vi "Storing Calibration Coefficients.vi"(11 "output cluster":T1) -> (1 "Array":dbl[](array[numeric]), 2 "Error":bool)   [LabVIEW 2016]
uses:
  Controls/Cal Refs.ctl
  Miscellaneous/Globals.vi
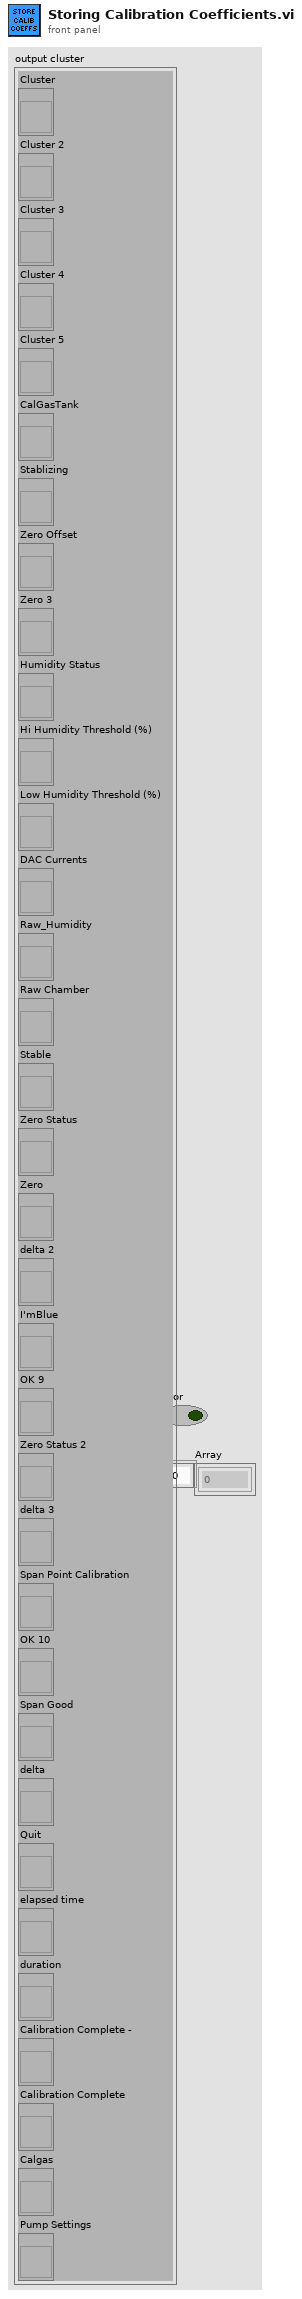
[diagram p1: front panel]
types:
  T1 = typedef "Cal Refs.ctl" = cluster{"Cluster":refnum<vi>, "Cluster 2":refnum<vi>, "Cluster 3":refnum<vi>, "Cluster 4":refnum<vi>, "Cluster 5":refnum<vi>, "CalGasTank":refnum<vi>, "Stablizing":refnum<vi>, "Zero Offset":refnum<vi>, "Zero 3":refnum<vi>, "Humidity Status":refnum<vi>, "Hi Humidity Threshold (%)":refnum<vi>, "Low Humidity Threshold (%)":refnum<vi>, "DAC Currents":refnum<vi>, "Raw_Humidity":refnum<vi>, "Raw Chamber":refnum<vi>, "Stable":refnum<vi>, "Zero Status":refnum<vi>, "Zero":refnum<vi>, "delta 2":refnum<vi>, "I'mBlue":refnum<vi>, "OK 9":refnum<vi>, "Zero Status 2":refnum<vi>, "delta 3":refnum<vi>, "Span Point Calibration":refnum<vi>, "OK 10":refnum<vi>, "Span Good":refnum<vi>, "delta":refnum<vi>, "Quit":refnum<vi>, "elapsed time":refnum<vi>, "duration":refnum<vi>, "Calibration Complete -":refnum<vi>, "Calibration Complete":refnum<vi>, "Calgas":refnum<vi>, "Pump Settings":refnum<vi>}
  T2 = typedef "Calibration Coefficients.ctl" = cluster{"CalFile Used":path, "TYPE":string, "DATE":string, "Humidity":sgl, "Chamber Temp":dbl, "CO2_calgas":dbl, "V_(RA,5mA)":dbl, "V_(RA,15mA)":dbl, "mI":dbl, "V_0d_ImA (actual)":dbl, "V_6d_ImA (actual)":dbl, "I_span":dbl, "DAC":u16, "A":dbl, "B":dbl, "C":dbl, "D":dbl, "V6d":dbl, "A'":dbl, "B'":dbl, "C'":dbl, "D'":dbl, "V0d":dbl, "CalDate":string, "CalTime":string, "duration":dbl, "Detector Channel":string, "a2":dbl, "a3":dbl, "a4":dbl, "a5":dbl, "b2":dbl, "c2":dbl, "b3":dbl, "c3":dbl, "b4":dbl, "c4":dbl, "b5":dbl, "c5":dbl, "a7":dbl, "a8":dbl, "a9":dbl, "a10":dbl, "b7":dbl, "b8":dbl, "b9":dbl, "b10":dbl, "c7":dbl, "c8":dbl, "c9":dbl, "c10":dbl, "cal_offs_adj":dbl, "cal_gain_adj":dbl, "C6d":dbl, "C0d":dbl, "Cal_currernt":dbl, "C2V":u16, "V2C":u16, "Zero Date":string, "Zero Time":string, "Number of Zeroes":u16, "V_(()d, average)":dbl, "V_offs ":dbl, "G_adj":dbl, "Pump Flow Rate":u16, "Zero Required? ":bool, "Calibrate Required?":bool, "cal_utc":dbl, "zero_utc":dbl, "Elapsed Time":dbl, "PCB":string, "m0":dbl, "b0":dbl}
  T3 = cluster{"CalFile Selected":path, "TYPE":string, "DATE":string, "C0FC2V":dbl[], "C6FC2V":dbl[], "V_0d(target)":dbl[], "V_6d(target)":dbl[], "V_span(target)":dbl[], "CHANNEL":string[], "Status":bool[], "BlueLED 2":bool[], "C2V":u8[], "A":dbl[], "B":dbl[], "C":dbl[], "D":dbl[], "V2C":u8[], "A'":dbl[], "B'":dbl[], "C'":dbl[], "D'":dbl[]}
  T4 = cluster{"CHANNEL 2":string[], "BlueLED":bool[], "V_RA(5mA)":dbl[], "V_RA(15mA)":dbl[], "mI":dbl[], "DAC scale":dbl[]}
  T5 = cluster{"CHANNEL 3":string[], "BlueLED 3":bool[], "V_RA(5mA) 2":dbl[], "V_RA(15mA) 2":dbl[], "mI 2":dbl[]}
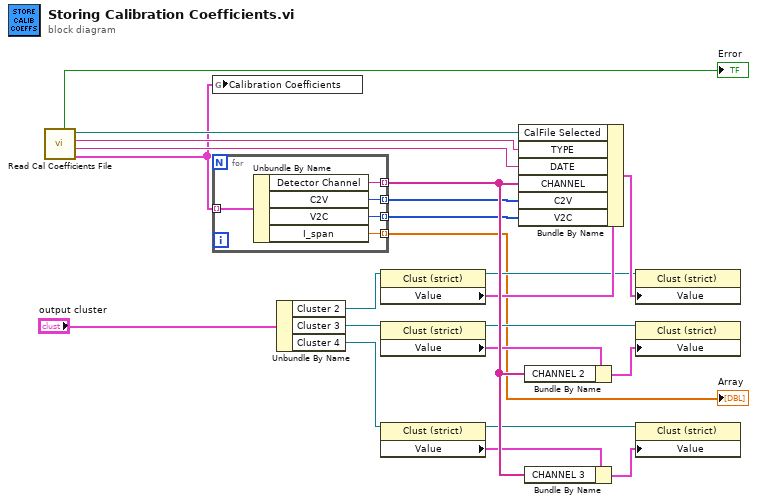
[diagram p0: block diagram]
diagram:
  n1 = call "Read Cal Coefficients File.vi"() -> ("Original Coefficients"=w1:T2[], "DATE"=w13:string, "TYPE"=w12:string, "CalFile Selected"=w11:path, "Error"=→"Error":bool)  [unwired: 6 in, 1 out]
  n2 = global write "Globals.vi" "Calibration Coefficients"(w1) -> ()
  n3 = for {
    tunnel: w1 -> [w27] mode=indexing
    tunnel: [w26] -> w7 mode=indexing
    tunnel: [w25] -> w15 mode=indexing
    tunnel: [w24] -> w14 mode=indexing
    tunnel: [w23] -> w22 mode=indexing
    n4 = Unbundle By Name(w27) -> ("Detector Channel"=w23:string, "C2V"=w24:u16, "V2C"=w25:u16, "I_span"=w26:dbl)
  }
  "Array" <- w7
  n5 = Unbundle By Name("output cluster") -> ("Cluster 2"=w4:refnum<vi>, "Cluster 3"=w3:refnum<vi>, "Cluster 4"=w2:refnum<vi>)
  n6 = property class="Clust (strict)"(reference=w4) -> (reference out=w8:refnum<vi>, "Value"=w9:T3)  [unwired: 1 in, 1 out]
  n7 = property class="Clust (strict)"(reference=w3) -> (reference out=w16:refnum<vi>, "Value"=w17:T4)  [unwired: 1 in, 1 out]
  n8 = property class="Clust (strict)"(reference=w2) -> (reference out=w20:refnum<vi>, "Value"=w21:T5)  [unwired: 1 in, 1 out]
  n9 = Bundle By Name(cluster=w9, "CalFile Selected"=w11, "TYPE"=w12, "DATE"=w13, "CHANNEL"=w22, "C2V"=w14, "V2C"=w15) -> (w10:T3)
  n10 = Bundle By Name(cluster=w17, "CHANNEL 2"=w22) -> (w18:T4)
  n11 = Bundle By Name(cluster=w21, "CHANNEL 3"=w22) -> (w19:T5)
  n12 = property class="Clust (strict)"(reference=w8, "Value"=w10) -> ()  [unwired: 1 in, 2 out]
  n13 = property class="Clust (strict)"(reference=w16, "Value"=w18) -> ()  [unwired: 1 in, 2 out]
  n14 = property class="Clust (strict)"(reference=w20, "Value"=w19) -> ()  [unwired: 1 in, 2 out]
